vi "ShiftRegisterTest.vi"() -> ()   [LabVIEW 2017]
panel:
  out "Out":dbl
  in  "Add":dbl
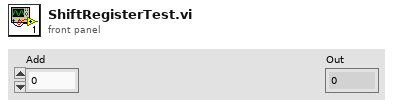
[diagram p1: front panel]
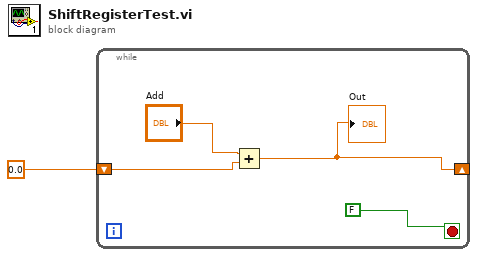
[diagram p0: block diagram]
diagram:
  n1 = while {
    shift-right: [w3] -> _
    shift-left: 0.0 -> [w4]
    stop <- FALSE stop-if-true
    n2 = Add(x="Add", y=w4) -> (x+y=w3:dbl)
    "Out" <- w3
  }
